vi "ConfigureMarkerEnabled.vi"(8 "error in (no error)":errorcluster, 11 "Keysight44xx in":refnum<class "Keysight44xx.lvclass">) -> (0 "error out":errorcluster, 3 "Keysight44xx out":refnum<class "Keysight44xx.lvclass">)   [LabVIEW 2018, in "SpecAnPlugins.lvlib" / "Keysight44xx.lvclass"]
doc: "This VI enables the active marker on the specified trace."
uses:
  Keysight44xx.lvclass
  C:/Users/ico/Documents/Projects/NistPluggableModules/SpecAn/SpecAnPlugins/SpecAnBaseClass/SpecAnBase.lvclass
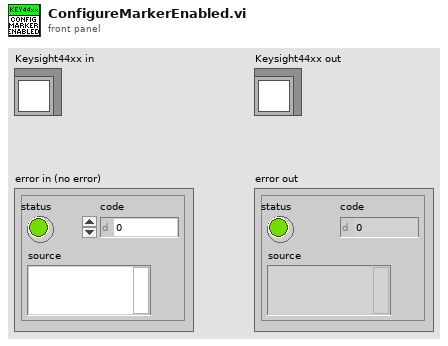
[diagram p1: front panel]
types:
  T1 = typedef "SpecAnPlugins.lvlib/SpecAnBase.lvclass/Acquisition.ctl" = cluster{"Handle":string, "Connected":bool, "Enabled":bool, "SweepModeContinuous":bool, "NumberOfSweeps":i32, "DetectorTypeAuto":bool, "DetectorType":i32, "VerticalScale":i32, "MaximumTime(seconds)":dbl}
  T2 = typedef "SpecAnPlugins.lvlib/SpecAnBase.lvclass/Markers.ctl" = cluster{"MarkerEnabled":bool, "MarkerThreshold":dbl, "PeakExcursion":dbl, "SignalTrackEnabled":bool, "MarkerPosition":dbl, "Instrument Setting (Frequency Center)":i32, "Marker search (Minimum)":i32, "ActiveMarker":string, "MarkerFrequencyCounter":bool, "FrequencyCounterResolution":dbl}
  T3 = typedef "SpecAnPlugins.lvlib/SpecAnBase.lvclass/Trace.ctl" = cluster{"TraceName":string, "TraceSize":i32, "TraceType":i32}[]
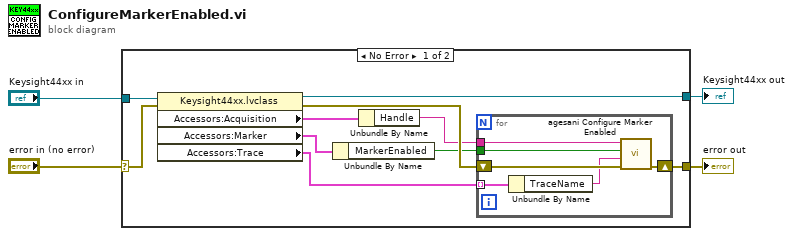
[diagram p0: block diagram]
diagram:
  n1 = case shown="No Error" "error in (no error)" {
    selector: "error in (no error)" -> [w13 w21]
    tunnel: [w10 w21] -> w3
    tunnel: "Keysight44xx in" -> [w14 w22]
    tunnel: [w12 w22] -> w1
    frame No Error {
      n2 = property class="Keysight44xx.lvclass"(reference=w14, error in=w13) -> (reference out=w12:refnum<class "Keysight44xx.lvclass">, error out=w11:errorcluster, "Accessors:Acquisition"=w8:T1, "Accessors:Marker"=w7:T2, "Accessors:Trace"=w5:T3)
      n3 = Unbundle By Name(w7) -> ("MarkerEnabled"=w6:bool)
      n4 = Unbundle By Name(w8) -> ("Handle"=w9:string)
      n5 = for {
        tunnel: w9 -> [w18]
        tunnel: w6 -> [w17]
        shift-right: [w19] -> w10
        shift-left: w11 -> [w20]
        tunnel: w5 -> [w16] mode=indexing
        n6 = Unbundle By Name(w16) -> ("TraceName"=w15:string)
        n7 = call <instrlib>:"agesani Configure Marker Enabled.vi"("error in (no error)"=w20, "marker trace name (\"\")"=w15, "marker enabled (Off)"=w17, "instrument handle"=w18) -> ("error out"=w19:errorcluster)  [unwired: 6 in, 1 out]
      }
    }
    frame Error {
    }
  }
  "error out" <- w3
  "Keysight44xx out" <- w1
